vi "smaract serial read hardware part.vi"(8 "error in (no error)":errorcluster, 10 "Get position commands":string[](array[string]), 11 "VISA Refnum in":refnum<visa-resource-name>) -> (0 "error out":errorcluster, 2 "Positions":i32[](array[numeric]), 3 "VISA Refnum out":refnum<visa-resource-name>)   [LabVIEW 2020, in "Smaract.lvclass"]
uses:
  Smaract.lvclass
  stop FGV control.ctl
  Smaract acquire fgv.ctl
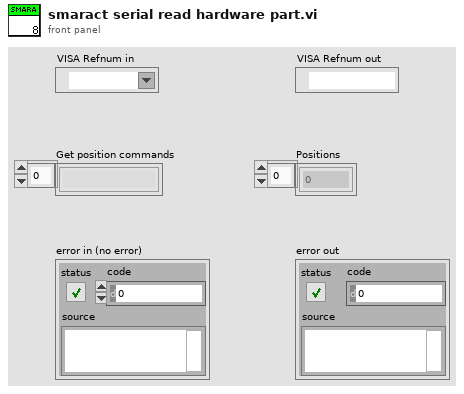
[diagram p1: front panel]
types:
  T1 = typedef "Smaract acquire fgv.ctl" = cluster{"busy":bool, "Positions":i32[]}
  T2 = typedef "stop FGV control.ctl" = enum16{"Clear", "Write", "Read"}
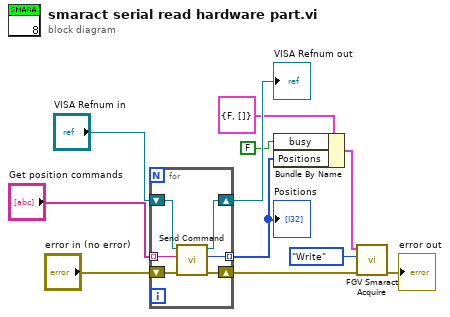
[diagram p0: block diagram]
diagram:
  n1 = for {
    tunnel: "Get position commands" -> [w17] mode=indexing
    tunnel: [w13] -> w2 mode=indexing
    shift-right: [w14] -> w6
    shift-left: "error in (no error)" -> [w16]
    shift-right: [w12] -> w8
    shift-left: "VISA Refnum in" -> [w15]
    n2 = call "Send Command.vi"("error in"=w16, "Command In"=w17, "Comport Smaract"=w15) -> ("error out"=w14:errorcluster, "Value"=w13:i32, "Comport Smaract out"=w12:refnum<visa-resource-name>)  [unwired: 6 in]
  }
  "Positions" <- w2
  "VISA Refnum out" <- w8
  n3 = Bundle By Name(cluster=T1 {"busy"=FALSE, "Positions"=[]} ("Smaract Acq Data"), "busy"=FALSE, "Positions"=w2) -> (w1:T1)
  n4 = call "FGV Smaract Acquire.vi"("error in"=w6, "Function"=stop_FGV_control."Write", "Smaract Acq Data"=w1) -> ("error out"=→"error out":errorcluster)  [unwired: 7 in, 1 out]
